vi "Obtain Default Broadcast Events.vi"(8 "error in (no error)":errorcluster) -> (0 "error out":errorcluster, 1 "Update Module Execution Status":refnum<user-event>, 2 "Error Reported":refnum<user-event>, 3 "Status Updated":refnum<user-event>, 4 "System Message":refnum<user-event>, 5 "Module Did Stop":refnum<user-event>)   [LabVIEW 2022 SP3, in "Dummy.lvlib"]
doc: "____\nHAMPEL SOFTWARE ENGINEERING v2.6.0 (2023-12-19 10:54)"
uses:
  Dummy.lvlib
  Get Module Execution Status Argument--cluster.ctl
  Status Updated Argument--cluster.ctl
  Error Reported Argument--cluster.ctl
  Stop Argument--cluster.ctl
  System Message Argument--cluster.ctl
  Libraries/hse-libraries/Source/hse-dqmh/Controls/System Message Source.ctl
  Libraries/hse-libraries/Source/hse-dqmh/hse-dqmh.lvlib
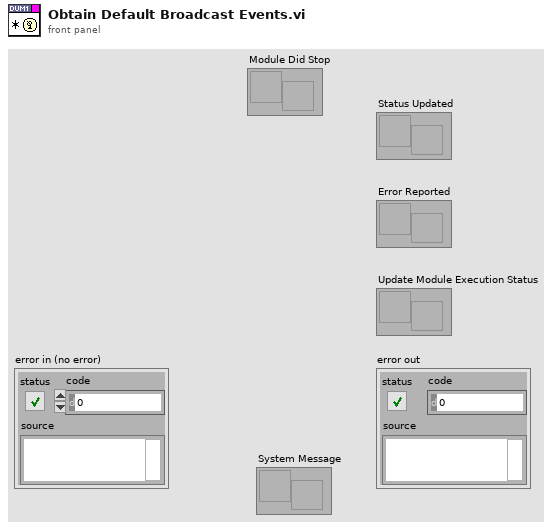
[diagram p1: front panel]
types:
  T1 = typedef "Dummy.lvlib/Broadcast Events--cluster.ctl" = cluster{"Module Did Init":refnum<user-event>, "Status Updated":refnum<user-event>, "Error Reported":refnum<user-event>, "Module Did Stop":refnum<user-event>, "Update Module Execution Status":refnum<user-event>, "System Message":refnum<user-event>}
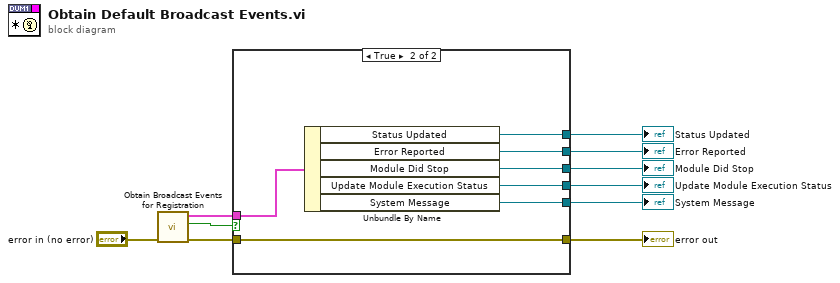
[diagram p0: block diagram]
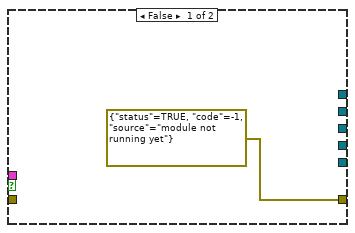
[diagram p2: hidden frame]
diagram:
  n1 = call "Obtain Broadcast Events for Registration.vi"("error in (no error)"="error in (no error)") -> ("error out"=w10:errorcluster, "Already running?"=w8:bool, "Dummy Broadcast Events"=w9:T1)  [unwired: 8 in]
  n2 = case shown="True" w8 {
    tunnel: w9 -> [_ w18]
    tunnel: [errorcluster {"status"=TRUE, "code"=-1, "source"="module not running yet"} ("error out") w17] -> w6
    tunnel: w10 -> [_ w17]
    tunnel: [_ w16] -> w4
    tunnel: [_ w15] -> w3
    tunnel: [_ w14] -> w2
    tunnel: [_ w13] -> w5
    tunnel: [_ w12] -> w1
    frame False {
    }
    frame True {
      n3 = Unbundle By Name(w18) -> ("Status Updated"=w16:refnum<user-event>, "Error Reported"=w15:refnum<user-event>, "Module Did Stop"=w14:refnum<user-event>, "Update Module Execution Status"=w13:refnum<user-event>, "System Message"=w12:refnum<user-event>)
    }
  }
  "error out" <- w6
  "Update Module Execution Status" <- w5
  "Status Updated" <- w4
  "Error Reported" <- w3
  "Module Did Stop" <- w2
  "System Message" <- w1
